vi "Check Download Complete.vi"(11 "data":T1[](array[typedef]) {"payload" format="%x"; "timestamp" format="%<%.7X\n%x>T"; "type" items=["CAN Data"=0, "CAN Remote"=1, "CAN Bus Error"=2, "CAN 2.0 Data"=8, "CAN FD Data"=16, "CAN FD+BRS Data"=24, "J1939 Data"=192, "Delay"=224, "Log Trigger"=225, "Start Trigger"=226]; "identifier" format="%x"}) -> (3 "Boolean":bool)   [LabVIEW 2018]
uses:
  <vilib>/xnet/xnet.llb/XNET Frame CAN.ctl
  <vilib>/xnet/xnet.llb/XNET Frame Type CAN.ctl
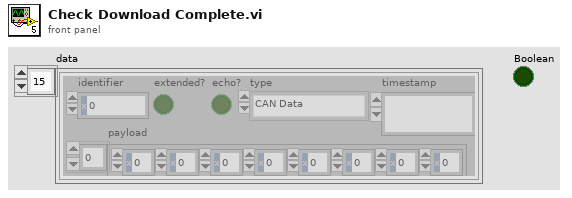
[diagram p1: front panel]
types:
  T1 = typedef "XNET Frame CAN.ctl" = cluster{"timestamp":timestamp, "payload":u8[], "identifier":u32, "type":T2, "extended?":bool, "echo?":bool}
  T2 = typedef "XNET Frame Type CAN.ctl" = u8
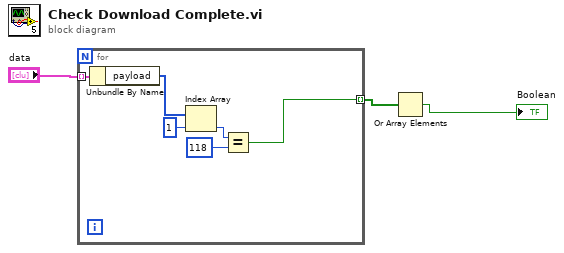
[diagram p0: block diagram]
diagram:
  n1 = for {
    tunnel: "data" -> [w9] mode=indexing
    tunnel: [w5] -> w2 mode=indexing
    n2 = Unbundle By Name(w9) -> ("payload"=w8:u8[])
    n3 = Index Array(array=w8, index=1) -> (element=w7:u8)
    n4 = Equal?(x=w7, y=u8 118) -> (x = y?=w5:bool)
  }
  n5 = Or Array Elements(Boolean array=w2) -> (logical OR=→"Boolean":bool)
